vi "Write Uml.vi"(8 "error in (no error)":errorcluster, 10 "Uml":string, 11 "Classes Overview in":refnum<class "Classes Overview.lvclass">) -> (0 "error out":errorcluster, 3 "Classes Overview out":refnum<class "Classes Overview.lvclass">)   [LabVIEW 2021, in "TAF Proj Document Type.lvlib" / "Classes Overview.lvclass"]
uses:
  <vilib>/Wovalab/AntiDoc/Document Type/Add-ons/LabVIEW TAF Project/Classes Overview/Classes Overview.lvclass
  <vilib>/Wovalab/AntiDoc/Document Type/Add-ons/LabVIEW TAF Project/Classes Overview/Classes Overview.lvclass/Classes Overview.ctl
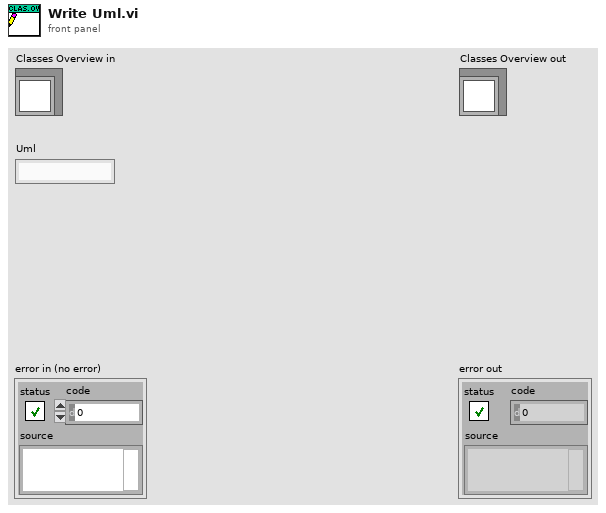
[diagram p1: front panel]
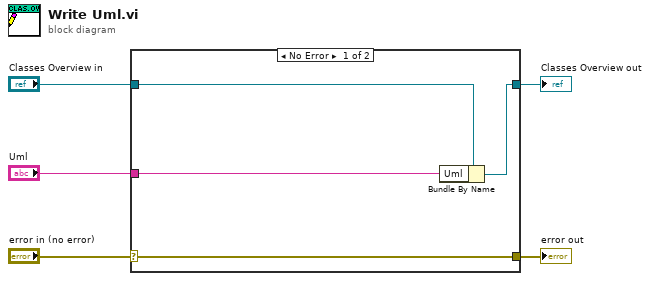
[diagram p0: block diagram]
diagram:
  n1 = case shown="No Error" "error in (no error)" {
    selector: "error in (no error)" -> [w9 w10]
    tunnel: [w9 w10] -> w4
    tunnel: [w7 w11] -> w2
    tunnel: "Classes Overview in" -> [w8 w11]
    tunnel: "Uml" -> [w6 _]
    frame No Error {
      n2 = Bundle By Name(cluster=w8, "Uml"=w6) -> (w7:refnum<class "Classes Overview.lvclass">)
    }
    frame Error {
    }
  }
  "error out" <- w4
  "Classes Overview out" <- w2
